vi "simulator 3.vi"() -> ()   [LabVIEW 2010]
uses:
  TCL-Target_Computer_Logging/TCL Global.vi
  TCL-Target_Computer_Logging/TCL Select Fragments/TCL Select Fragments 1frag1criterium.vi
panel:
  in  "active baseline file":path
  in  "signal":string
  in  "simulate QCA signal":bool
  in  "period (s)":dbl
  in  "initiate events":bool
  in  "stop":bool
  out "next time to simulate":timestamp
  out "next event to simulate":u64
  out "last time processed":timestamp
  out "last time simulated":timestamp
  out "last event processed":u64
  out "last event simulated":u64
  in  "reset map":bool
  in  "first time to simulate":timestamp
  in  "first event to simulate":u64
  in  "primary key":string
  in  "simulation file":path
  in  "modules":T1(array[cluster])
  # "This VI allows one to simulate inputs from various PDP modules. When the enabled modules receive a GenEvent= message, they send the specified fragments to the Target Event Builder (TEB). The VI can send manually entered values for these fragments or read them sequentially from a simulus file, which should have the same format as an event file (one can simulate previous runs by loading in old event files).\n\nTo use this simulator:\n\n1. Configure the modules you want to simulate at right.\n2. In value mode, enter fragment names and their corresponding simulated values. In file mode, enter fragment names and their corresponding field names for file lookup. Repeat for each module.\n3. If using file mode, choose your data file (same format as event files) and select the first event number to simulate. By default, simulation will start with the first event in the file.\n4. Run PDP. Modules will respond to GenEvent= messages with the listed fragments.\n\nTo initiate TEB events periodically (a job that QCA normally handles), use the controls above. To simulate QCA signals, use the controls at top right."
  # "value"
  # "file"
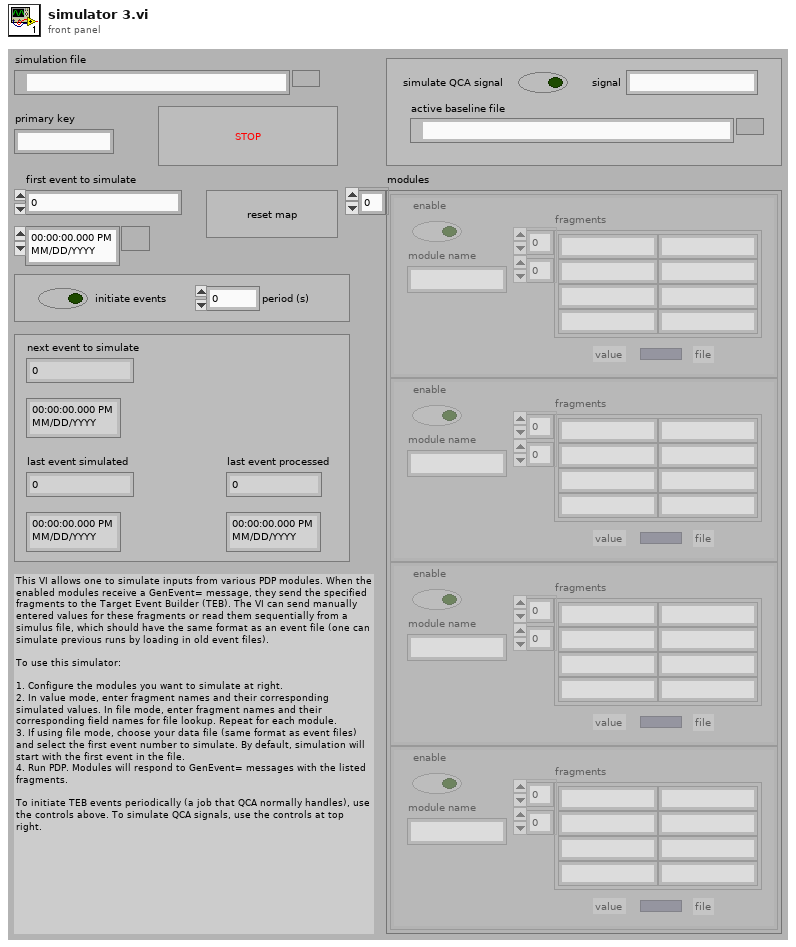
[diagram p1: front panel]
types:
  T1 = cluster{"enable":bool, "module name":string, "fragments":string[][], "file":bool}[]
  T2 = enum16{"reset map", "generate qca signal", "listen for messages", "stop"}
  T3 = cluster{enum16{"reset map", "generate qca signal", "listen for messages", "stop"}, u64}
  T4 = cluster{"fragment":string, "values":string[], "operator":string}
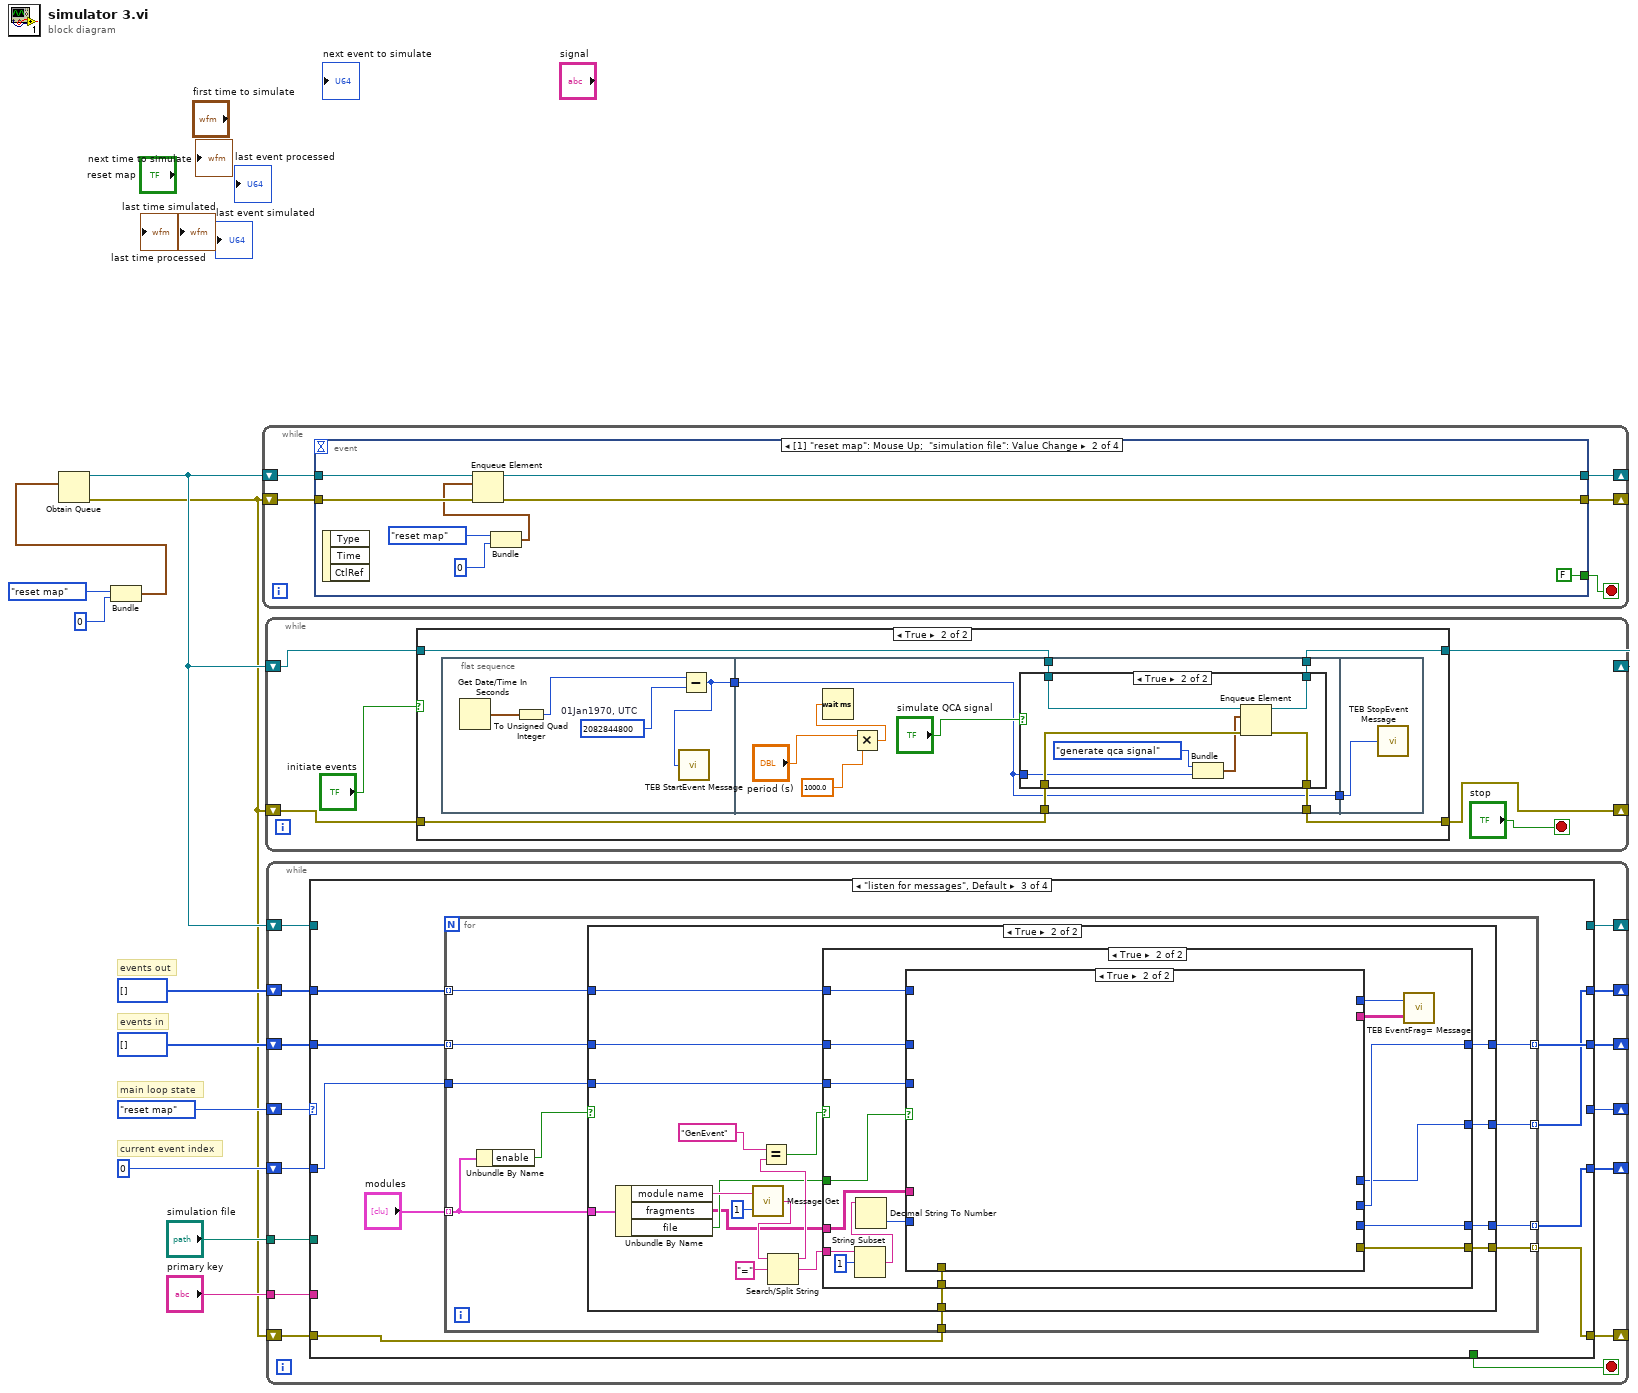
[diagram p0: block diagram]
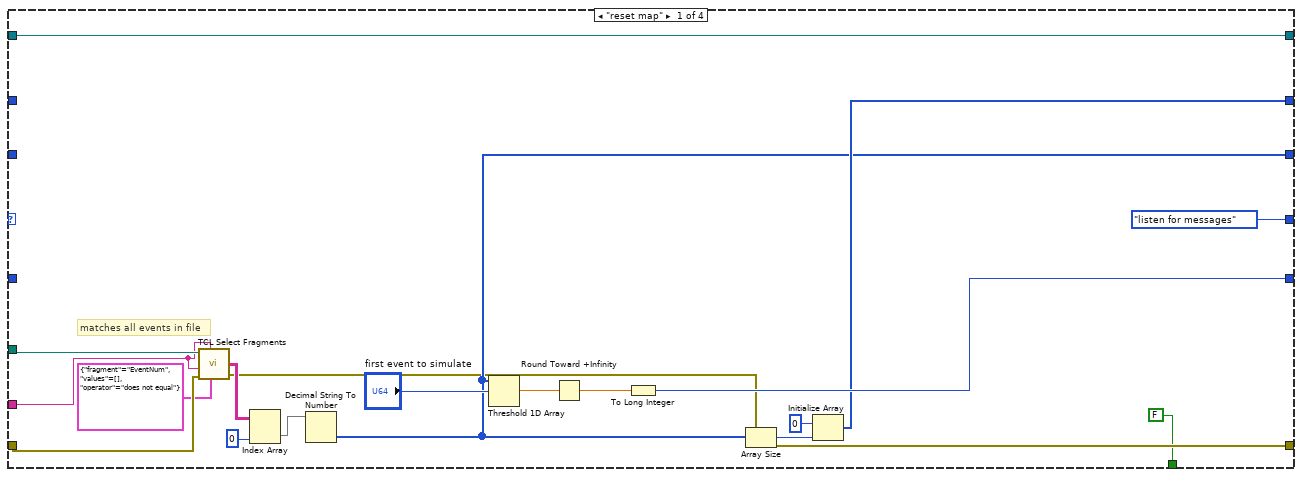
[diagram p2: hidden frame]
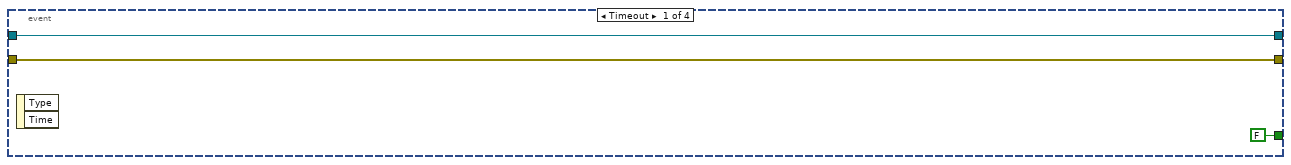
[diagram p10: hidden frame]
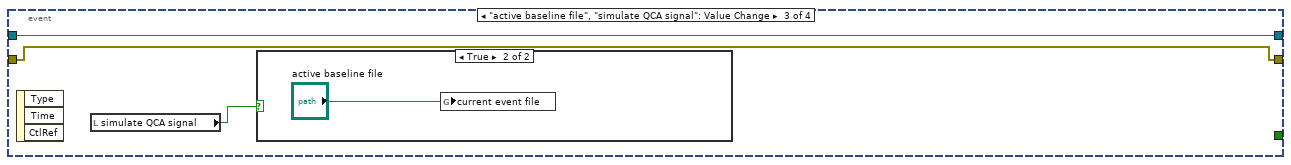
[diagram p11: hidden frame]
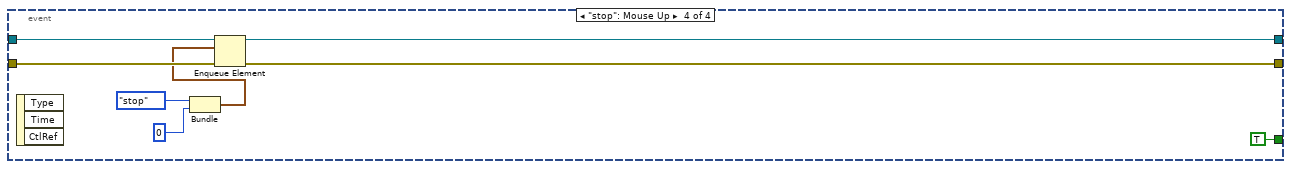
[diagram p13: hidden frame]
diagram:
  # "current event index"
  # "events out"
  # "events in"
  # "main loop state"
  n1 = Bundle(T2."reset map", u64 0) -> (w4:T3)  [unwired: 1 in]
  n2 = Obtain Queue(element data type=w4) -> (queue out=w8:refnum<queue>, error out=w1:errorcluster)  [unwired: 4 in, 1 out]
  n3 = while {
    shift-right: [w13] -> _
    shift-left: w8 -> [w16]
    shift-right: [w14] -> _
    shift-left: w1 -> [w15]
    stop <- w12 stop-if-true
    n4 = event shown="[1] \"reset map\": Mouse Up;  \"simulation file\": Value Change" {
      selector: _ -> [_ _ _ _]
      dyn-events: _ -> [_ _ _ _]
      timeout: _ -> [_ _ _ _]
      tunnel: w16 -> [w18 w27 w28 w38]
      tunnel: w15 -> [w19 w26 w29 w37]
      tunnel: [w19 w25 w29 w36] -> w14
      tunnel: [w18 w24 w28 w35] -> w13
      tunnel: [FALSE FALSE _ TRUE] -> w12
      event Timeout {
        n5 = event-data() -> ()  [unwired: 1 in, 2 out]
      }
      event "reset map": Mouse Up; "simulation file": Value Change {
        n6 = event-data() -> ()  [unwired: 1 in, 3 out]
        n7 = Bundle(T2."reset map", u64 0) -> (w21:T3)  [unwired: 1 in]
        n8 = Enqueue Element(queue=w27, element=w21, error in (no error)=w26) -> (queue out=w24:refnum<queue>, error out=w25:errorcluster)  [unwired: 1 in, 1 out]
      }
      event "active baseline file", "simulate QCA signal": Value Change {
        n9 = event-data() -> ()  [unwired: 1 in, 3 out]
        n10 = local read "simulate QCA signal"() -> (w30:bool)
        n11 = case shown="True" w30 {
          frame False {
          }
          frame True {
            n12 = global write "TCL Global.vi" "current event file"("active baseline file") -> ()
          }
        }
      }
      event "stop": Mouse Up {
        n13 = event-data() -> ()  [unwired: 1 in, 3 out]
        n14 = Bundle(T2."stop", u64 0) -> (w32:T3)  [unwired: 1 in]
        n15 = Enqueue Element(queue=w38, element=w32, error in (no error)=w37) -> (queue out=w35:refnum<queue>, error out=w36:errorcluster)  [unwired: 1 in, 1 out]
      }
    }
  }
  n16 = while {
    shift-right: [w40] -> _
    shift-left: w8 -> [w43]
    shift-right: [w41] -> _
    shift-left: w1 -> [w42]
    stop <- "stop" stop-if-true
    n17 = case shown="True" "initiate events" {
      tunnel: w43 -> [w47 w53]
      tunnel: w42 -> [w46 w52]
      tunnel: [w46 w51] -> w41
      tunnel: [w47 w50] -> w40
      frame False {
      }
      frame True {
        n18 = flat-sequence {
          tunnel: [w54] -> w49
          tunnel: w53 -> [w62]
          tunnel: w52 -> [w61]
          tunnel: [w60] -> w51
          tunnel: [w59] -> w50
          tunnel: w49 -> [w58]
          tunnel: [w58] -> w48
          tunnel: w48 -> [w76]
          frame #0 {
            w55 = u64 2082844800  # 01Jan1970, UTC
            n19 = Get Date/Time In Seconds() -> (seconds since 1Jan1904=w57:timestamp)
            n20 = To Unsigned Quad Integer(1:w57) -> (0:w56:u64)
            n21 = Subtract(x=w56, y=w55) -> (x-y=w54:u64)
            n22 = call "TEB StartEvent Message.vi"("Event Number"=w54) -> ()
          }
          frame #1 {
            n23 = Multiply(x="period (s)", y=1000.0) -> (x*y=w66:dbl)
            n24 = Wait (ms)(milliseconds to wait=w66) -> ()  [unwired: 1 out]
            n25 = case shown="True" "simulate QCA signal" {
              tunnel: w62 -> [w67 w75]
              tunnel: w61 -> [w68 w74]
              tunnel: [w68 w73] -> w60
              tunnel: [w67 w72] -> w59
              tunnel: w58 -> [_ w69]
              frame False {
              }
              frame True {
                n26 = Bundle(T2."generate qca signal", w69) -> (w71:T3)  [unwired: 1 in]
                n27 = Enqueue Element(queue=w75, element=w71, error in (no error)=w74) -> (queue out=w72:refnum<queue>, error out=w73:errorcluster)  [unwired: 1 in, 1 out]
              }
            }
          }
          frame #2 {
            n28 = call "TEB StopEvent Message.vi"("Event Number"=w76) -> ()
          }
        }
      }
    }
  }
  n29 = while {
    shift-right: [w85] -> _
    shift-left: T2."reset map" -> [w91]
    shift-right: [w79] -> _
    shift-left: u64[] [] -> [w89]
    shift-right: [w80] -> _
    shift-left: u64[] [] -> [w90]
    shift-right: [w86] -> _
    shift-left: w8 -> [w88]
    tunnel: "simulation file" -> [w84]
    tunnel: "primary key" -> [w83]
    shift-right: [w78] -> _
    shift-left: w1 -> [w82]
    shift-right: [w81] -> _
    shift-left: 0 -> [w87]
    stop <- w77 stop-if-true
    n30 = case shown="\"listen for messages\", Default" w91 {
      tunnel: w90 -> [_ _ w114 _]
      tunnel: w89 -> [_ _ w113 _]
      tunnel: w88 -> [w110 _ _ _]
      tunnel: w87 -> [_ _ w112 _]
      tunnel: [w110 _ _ _] -> w86
      tunnel: [T2."listen for messages" _ _ _] -> w85
      tunnel: w84 -> [w108 _ _ _]
      tunnel: w83 -> [w105 _ _ _]
      tunnel: w82 -> [w107 _ w111 _]
      tunnel: [w96 _ w117 _] -> w81
      tunnel: [w95 _ w115 _] -> w80
      tunnel: [w94 _ w116 _] -> w79
      tunnel: [w93 _ w118 _] -> w78
      tunnel: [FALSE _ _ _] -> w77
      frame "reset map" {
        # "matches all events in file"
        n31 = call-poly "TCL Select Fragments.vi"("event file"=w108, "fragment"=w105, "primary key"=w105, "criterium"=T4 {"fragment"="EventNum", "values"=[], "operator"="does not equal"}, "error in (no error)"=w107) -> ("matches"=w101:string[][], "error out"=w93:errorcluster)  [unwired: 1 in, 1 out]
        n32 = Index Array(array=w101, index (col)=0 ("disabled index (col)")) -> (element=w99:string[])  [unwired: 1 in]
        n33 = Decimal String To Number(string=w99) -> (number=w94:i32[])  [unwired: 2 in, 1 out]
        n34 = Threshold 1D Array(2:"first event to simulate", 3:w94) -> (0:w103:dbl)  [unwired: 1 in]
        n35 = Round Toward +Infinity(x=w103) -> (ceil(x): smallest int >= x=w102:dbl)
        n36 = To Long Integer(number=w102) -> (32bit integer=w96:i32)
        n37 = Array Size(array=w94) -> (size(s)=w98:i32)
        n38 = Initialize Array(0 ("String"), w98) -> (w95:i32[])
      }
      frame "generate qca signal" {
      }
      frame "listen for messages", Default {
        n39 = for {
          tunnel: "modules" -> [w128] mode=indexing
          tunnel: [w127] -> w118 mode=indexing
          tunnel: [w126] -> w117 mode=indexing
          tunnel: [w125] -> w116 mode=indexing
          tunnel: [w124] -> w115 mode=indexing
          tunnel: w114 -> [w123] mode=indexing
          tunnel: w113 -> [w122] mode=indexing
          tunnel: w112 -> [w121]
          tunnel: w111 -> [w120]
          n40 = Unbundle By Name(w128) -> ("enable"=w129:bool)
          n41 = case shown="True" w129 {
            tunnel: w128 -> [_ w148]
            tunnel: [_ w137] -> w127
            tunnel: [_ w136] -> w126
            tunnel: [_ w135] -> w125
            tunnel: [_ w134] -> w124
            tunnel: w123 -> [_ w133]
            tunnel: w122 -> [_ w132]
            tunnel: w121 -> [_ w131]
            tunnel: w120 -> [_ w130]
            frame False {
            }
            frame True {
              n42 = Unbundle By Name(w148) -> ("module name"=w147:string, "fragments"=w138:string[][], "file"=w139:bool)
              n43 = call "Message Get.vi"("Timeout ms (-1)"=1, "Module"=w147) -> ("data out"=w144:string)
              n44 = Search/Split String(string=w144, search string/char (-)="=") -> (substring before match=w142:string, match + rest of string=w140:string)  [unwired: 1 in, 1 out]
              n45 = Equal?(x="GenEvent", y=w142) -> (x = y?=w141:bool)
              n46 = case shown="True" w141 {
                tunnel: w140 -> [_ w163]
                tunnel: w139 -> [_ w161]
                tunnel: w138 -> [_ w157]
                tunnel: [_ w156] -> w137
                tunnel: [_ w155] -> w136
                tunnel: [_ w154] -> w135
                tunnel: [_ w153] -> w134
                tunnel: w133 -> [_ w152]
                tunnel: w132 -> [_ w151]
                tunnel: w131 -> [_ w150]
                tunnel: w130 -> [_ w149]
                frame False {
                }
                frame True {
                  n47 = String Subset(string=w163, offset (0)=1) -> (substring=w162:string)  [unwired: 1 in]
                  n48 = Decimal String To Number(string=w162) -> (number=w158:i32)  [unwired: 2 in, 1 out]
                  n49 = case shown="True" w161 {
                    tunnel: [w170 _] -> w160
                    tunnel: [w169 _] -> w159
                    tunnel: w158 -> [w170 _]
                    tunnel: w157 -> [w169 _]
                    tunnel: [w168 _] -> w156
                    tunnel: [w167 _] -> w155
                    tunnel: [w166 _] -> w154
                    tunnel: [w165 _] -> w153
                    tunnel: w152 -> [w165 _]
                    tunnel: w151 -> [w166 _]
                    tunnel: w150 -> [w167 _]
                    tunnel: w149 -> [w168 _]
                    frame False {
                    }
                    frame True {
                    }
                  }
                  n50 = call "TEB EventFrag= Message.vi"("Event Fragment(s)"=w159, "Event Number"=w160) -> ()
                }
              }
            }
          }
        }
      }
      frame "stop" {
      }
    }
  }
